vi "Get Exposure Mode.vi"(8 "error in (no error)":errorcluster, 11 "Camera in":refnum<class "Camera.lvclass">) -> (0 "error out":errorcluster, 2 "Exposure Mode":T1, 3 "Camera":refnum<class "Camera.lvclass">)   [LabVIEW 2020, in "Camera.lvclass"]
uses:
  Camera.lvclass
  Exposure Mode.ctl
  Camera.lvclass/Camera.ctl
  1d0181f0-64a9-471c-9d08-be33338c9a07.vi
  84d87f68-00df-4f07-8889-951d30b90fde.vi
  GetSetStringValue.vi
  Check Not Disconnected.vi
  <vilib>/Comparison/Equal/Equal Functor/Equal Functor.lvclass
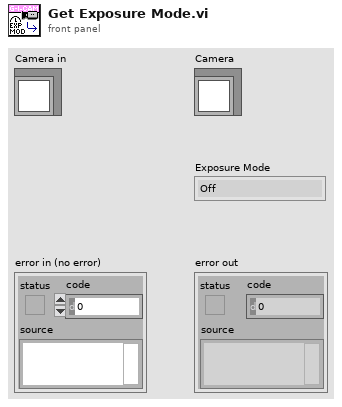
[diagram p1: front panel]
types:
  T1 = typedef "Camera.lvclass/Exposure Mode.ctl" = enum8{"Off", "Timed", "Trigger Width", "Trigger Controller"}
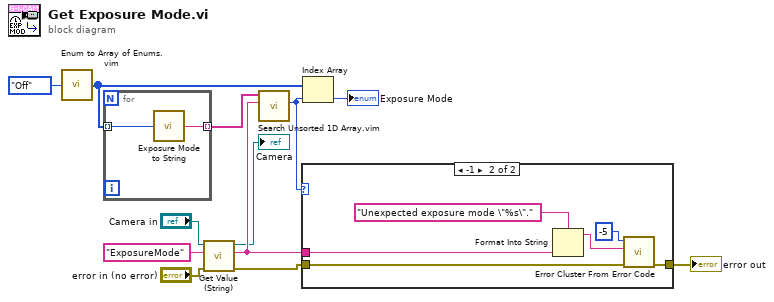
[diagram p0: block diagram]
diagram:
  n1 = call "Enum to Array of Enums.vim"("enum"=Exposure_Mode."Off" ("Exposure Mode")) -> ("array of enums"=w8:T1[])
  n2 = for {
    tunnel: w8 -> [w13] mode=indexing
    tunnel: [w14] -> w9 mode=indexing
    n3 = call "Exposure Mode to String.vi"("Exp Mode"=w13) -> ("String"=w14:string)
  }
  n4 = call "Get Value (String).vi"("error in (no error)"="error in (no error)", "Name"="ExposureMode", "Camera in"="Camera in") -> ("error out"=w3:errorcluster, "Value"=w2:string, "Camera"=→"Camera":refnum<class "Camera.lvclass">)  [unwired: 6 in]
  n5 = call "Search Unsorted 1D Array.vim"("element"=w2, "unsorted 1D array"=w9) -> ("index of element"=w5:i32)  [unwired: 9 in]
  n6 = case shown="-1" w5 {
    tunnel: [w15 w21] -> w4
    tunnel: w3 -> [w15 w20]
    tunnel: w2 -> [_ w16]
    frame Default {
    }
    frame -1 {
      n7 = Format Into String(format string="Unexpected exposure mode \"%s\"." ("error message (\"\")"), w16) -> (resulting string=w18:string)  [unwired: 2 in, 1 out]
      n8 = call <vilib>:"Error Cluster From Error Code.vi"("error in (no error)"=w20, "error message (\"\")"=w18, "error code (0)"=-5) -> ("error out"=w21:errorcluster)  [unwired: 6 in]
    }
  }
  "error out" <- w4
  n9 = Index Array(array=w8, index=w5) -> (element=→"Exposure Mode":T1)
